vi "温湿度上位机.vi"() -> ()   [LabVIEW 2023]
uses:
  <vilib>/Instr/_visa.llb/VISA Configure Serial Port (Instr).vi
panel:
  out "传输次数":dbl
  out "湿度计":dbl(slide) scale=0.0..100.0
  out "温度计":dbl(slide) scale=0.0..100.0
  out "EE":string
  out "FF":string
  out "温度":dbl
  out "湿度":dbl
  out "读取字节数":u32
  out "VISA资源名称输出":refnum<visa-resource-name>
  out "read buffer":string
  out "send flag":bool
  in  "波特率":u64(ring) items=["9600"=9600, "115200"=115200]
  in  "停止":bool
  out "枚举":T1
  out "Serial state":bool
  in  "serial":refnum<visa-resource-name> caption="端口号"
  in  "打开串口":bool
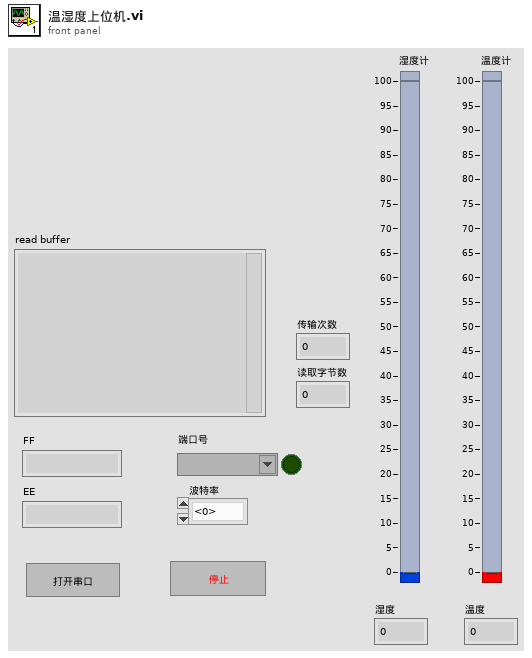
[diagram p1: front panel]
types:
  T1 = typedef "状态机.ctl" = enum16{"Init", "Wait", "GetData", "Send", "Deal", "Exit"}
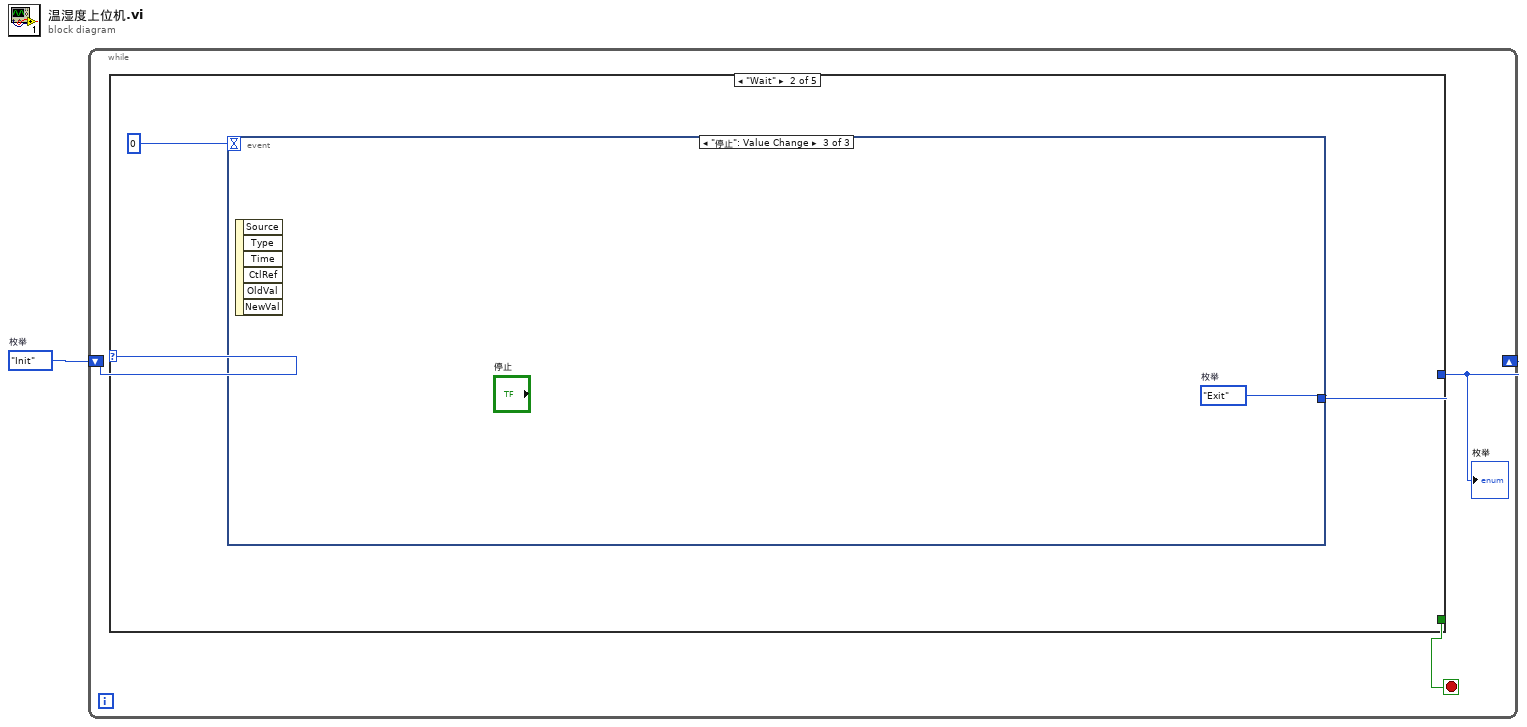
[diagram p0: block diagram]
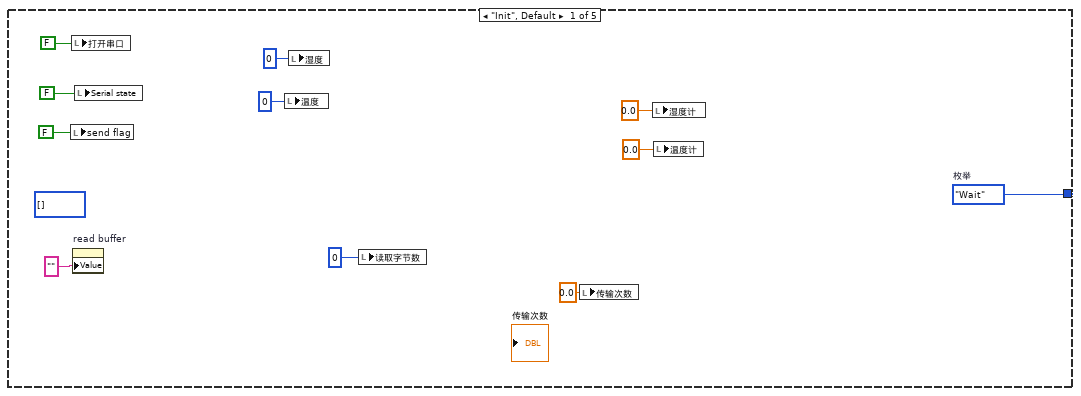
[diagram p2: hidden frame]
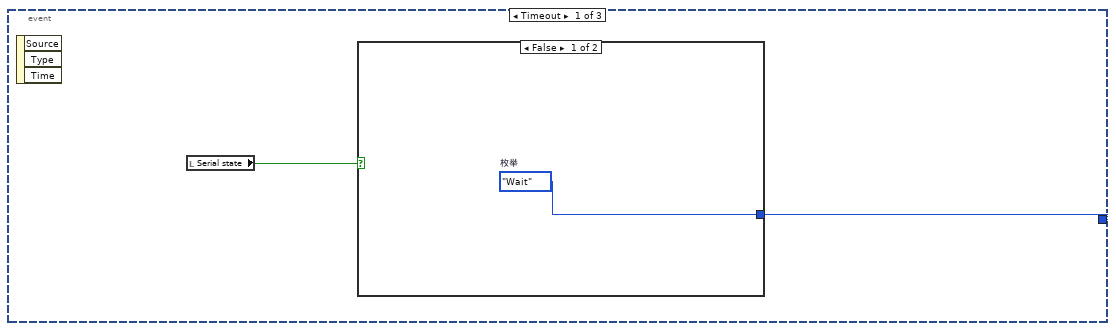
[diagram p3: hidden frame]
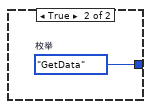
[diagram p4: hidden frame]
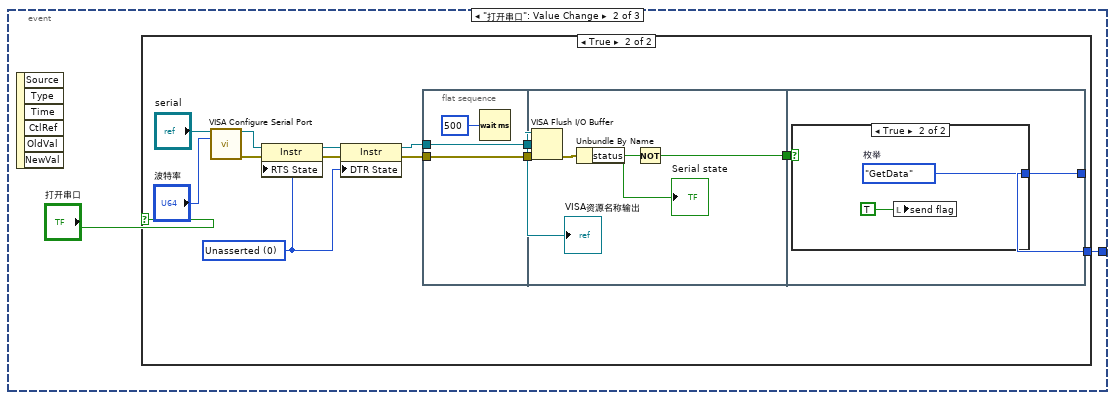
[diagram p5: hidden frame]
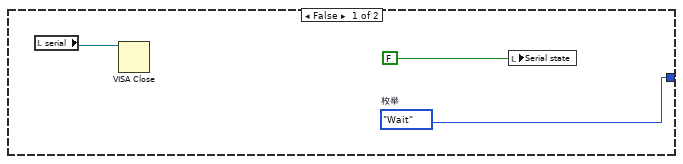
[diagram p6: hidden frame]
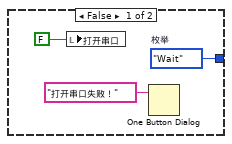
[diagram p7: hidden frame]
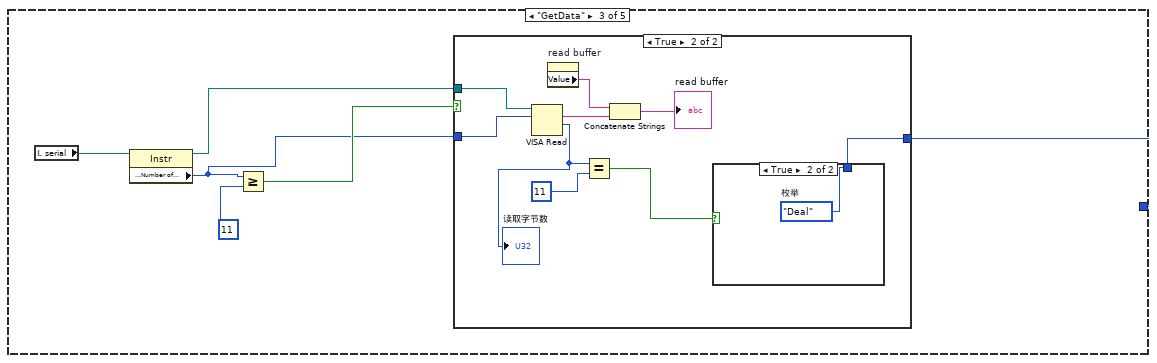
[diagram p8: hidden frame]
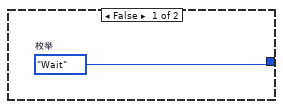
[diagram p9: hidden frame]
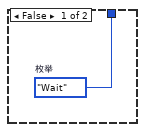
[diagram p10: hidden frame]
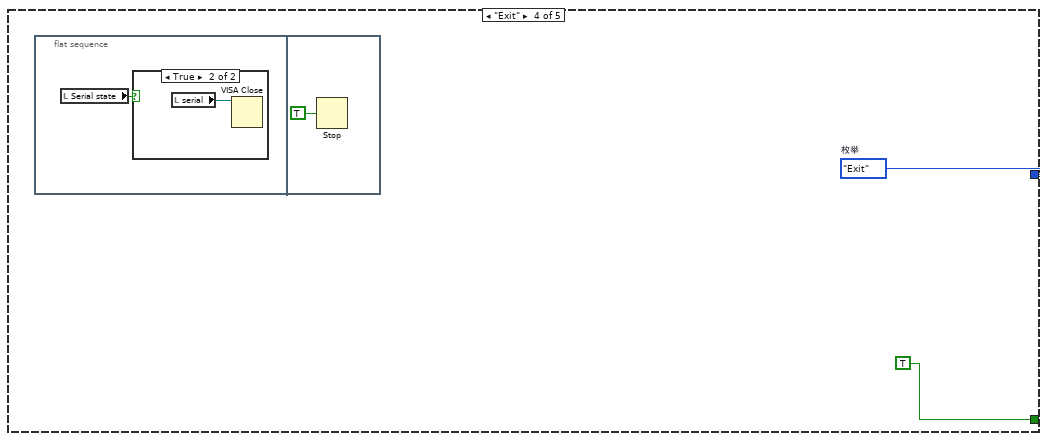
[diagram p11: hidden frame]
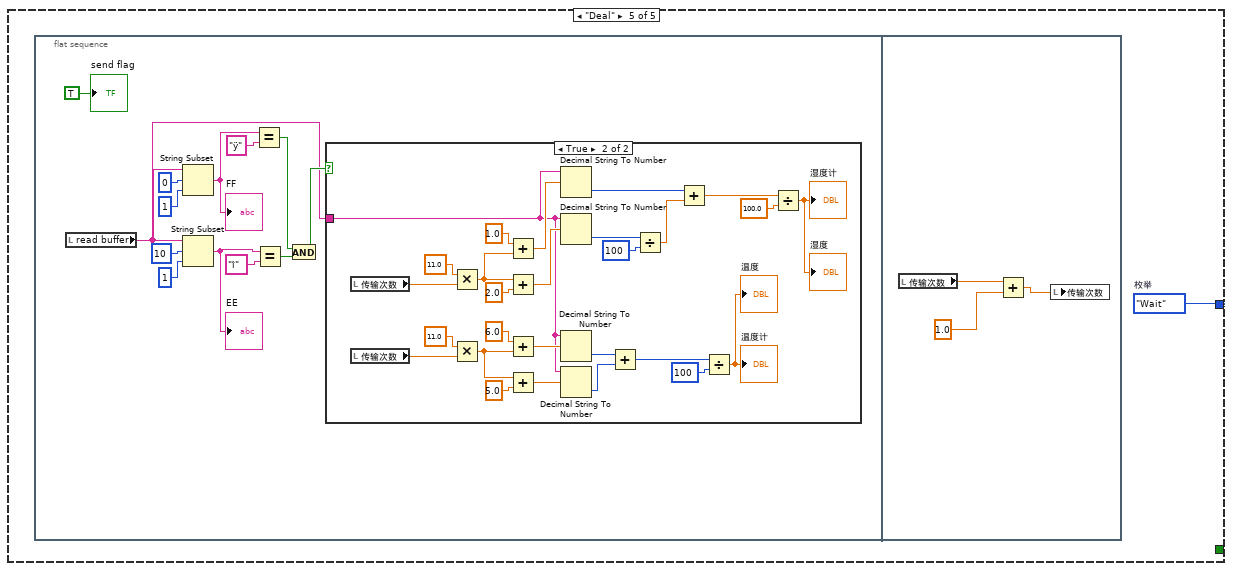
[diagram p13: hidden frame]
diagram:
  w1 = 状态机."Init"  # 枚举
  n1 = while {
    shift-right: [w3] -> _
    shift-left: w1 -> [w4]
    stop <- w2 stop-if-true
    n2 = case shown="\"Wait\"" w4 {
      tunnel: [w13 w16 w60 w76 w80] -> w3
      tunnel: [_ _ _ TRUE _] -> w2
      frame "Init", Default {
        (unwired) u32[] [] ("历史数据")
        w13 = 状态机."Wait"  # 枚举
        n3 = local write "send flag"(FALSE ("send flag")) -> ()
        n4 = local write "打开串口"(FALSE ("打开串口")) -> ()
        n5 = property on="read buffer" class="Str"("Value"="" ("read buffer")) -> ()  [unwired: 2 in, 2 out]
        n6 = local write "Serial state"(FALSE ("布尔")) -> ()
        n7 = local write "温度"(0 ("温度")) -> ()
        n8 = local write "湿度"(0 ("湿度")) -> ()
        n9 = local write "读取字节数"(u32 0 ("读取字节数")) -> ()
        n10 = local write "传输次数"(0.0 ("数值")) -> ()
        n11 = local write "湿度计"(0.0 ("湿度计")) -> ()
        n12 = local write "温度计"(0.0 ("温度计")) -> ()
      }
      frame "Wait" {
        n13 = event shown="[2] \"停止\": Value Change" {
          selector: _ -> [_ _ _]
          dyn-events: _ -> [_ _ _]
          timeout: 0 -> [_ _ _]
          tunnel: [w18 w22 w56] -> w16
          event Timeout {
            n14 = event-data() -> ()  [unwired: 1 in, 3 out]
            n15 = local read "Serial state"() -> (w19:bool)
            n16 = case shown="False" w19 {
              tunnel: [w20 w21] -> w18
              frame False {
                w20 = 状态机."Wait"  # 枚举
              }
              frame True {
                w21 = 状态机."GetData"  # 枚举
              }
            }
          }
          event "打开串口": Value Change {
            n17 = event-data() -> ()  [unwired: 1 in, 6 out]
            n18 = case shown="True" "打开串口" {
              tunnel: [w25 w27] -> w22
              frame False {
                w25 = 状态机."Wait"  # 枚举
                n19 = local read "serial"() -> (w24:refnum<visa-resource-name>)
                n20 = VISA Close(VISA resource name=w24) -> ()  [unwired: 1 in, 1 out]
                n21 = local write "Serial state"(FALSE ("布尔")) -> ()
              }
              frame True {
                w35 = i16 0 items=["Unknown"=-1, "Unasserted"=0, "Asserted"=1] ("Serial Settings:Modem Line Settings:Line DTR State")
                n22 = call-poly "VISA Configure Serial Port"("VISA resource name"="serial", "baud rate (9600)"="波特率") -> ("VISA resource name out"=w34:refnum<visa-resource-name>, "error out"=w33:errorcluster)  [unwired: 12 in]
                n23 = property class="Instr"(reference=w34, error in=w33, "RTS State"=w35) -> (reference out=w36:refnum<visa-resource-name>, error out=w37:errorcluster)
                n24 = property class="Instr"(reference=w36, error in=w37, "DTR State"=w35) -> (reference out=w32:refnum<visa-resource-name>, error out=w29:errorcluster)
                n25 = flat-sequence {
                  tunnel: w32 -> [w41]
                  tunnel: [w41] -> w31
                  tunnel: [w40] -> w30
                  tunnel: w29 -> [w40]
                  tunnel: w31 -> [w48]
                  tunnel: w30 -> [w44]
                  tunnel: [w45] -> w28
                  tunnel: w28 -> [w50]
                  tunnel: [w49] -> w27
                  frame #0 {
                    n26 = Wait (ms)(milliseconds to wait=u32 500 ("等待时间（毫秒）")) -> ()  [unwired: 1 out]
                  }
                  frame #1 {
                    n27 = VISA Flush I/O Buffer(VISA resource name=w48, error in (no error)=w44) -> (VISA resource name out=→"VISA资源名称输出":refnum<visa-resource-name>, error out=w46:errorcluster)  [unwired: 1 in]
                    n28 = Unbundle By Name(w46) -> ("status"=w47:bool)
                    n29 = Not(x=w47) -> (.not. x?=w45:bool)
                    "Serial state" <- w45
                  }
                  frame #2 {
                    n30 = case shown="True" w50 {
                      tunnel: [w51 w55] -> w49
                      frame False {
                        w51 = 状态机."Wait"  # 枚举
                        n31 = local write "打开串口"(FALSE ("打开串口")) -> ()
                        n32 = One Button Dialog(message="打开串口失败！" ("消息")) -> ()  [unwired: 1 in, 1 out]
                      }
                      frame True {
                        w55 = 状态机."GetData"  # 枚举
                        n33 = local write "send flag"(TRUE ("send flag")) -> ()
                      }
                    }
                  }
                }
              }
            }
          }
          event "停止": Value Change {
            w56 = 状态机."Exit"  # 枚举
            n34 = event-data() -> ()  [unwired: 1 in, 6 out]
          }
        }
      }
      frame "GetData" {
        n35 = local read "serial"() -> (w62:refnum<visa-resource-name>)
        n36 = property class="Instr"(reference=w62) -> (reference out=w61:refnum<visa-resource-name>, "Serial Settings:Number of Bytes at Serial Port"=w58:u32)  [unwired: 1 in, 1 out]
        n37 = Greater Or Equal?(x=w58, y=u32 11) -> (x >= y?=w59:bool)
        n38 = case shown="True" w59 {
          tunnel: w61 -> [_ w72]
          tunnel: w58 -> [_ w71]
          tunnel: [w63 w67] -> w60
          frame False {
            w63 = 状态机."Wait"  # 枚举
          }
          frame True {
            n39 = VISA Read(VISA resource name=w72, byte count=w71) -> (read buffer=w66:string, return count=w70:u32)  [unwired: 1 in, 2 out]
            "读取字节数" <- w70
            n40 = property on="read buffer" class="Str"() -> ("Value"=w64:string)  [unwired: 2 in, 2 out]
            n41 = Equal?(x=w70, y=u32 11) -> (x = y?=w68:bool)
            n42 = Concatenate Strings(w64, w66) -> (→"read buffer":string)
            n43 = case shown="True" w68 {
              tunnel: [w73 w74] -> w67
              frame False {
                w73 = 状态机."Wait"  # 枚举
              }
              frame True {
                w74 = 状态机."Deal"  # 枚举
              }
            }
          }
        }
      }
      frame "Exit" {
        w76 = 状态机."Exit"  # 枚举
        n44 = flat-sequence {
          frame #0 {
            n45 = local read "Serial state"() -> (w77:bool)
            n46 = case shown="True" w77 {
              frame False {
              }
              frame True {
                n47 = local read "serial"() -> (w78:refnum<visa-resource-name>)
                n48 = VISA Close(VISA resource name=w78) -> ()  [unwired: 1 in, 1 out]
              }
            }
          }
          frame #1 {
            n49 = Stop(stop? (T)=TRUE ("停止？(T)")) -> ()
          }
        }
      }
      frame "Deal" {
        w80 = 状态机."Wait"  # 枚举
        n50 = flat-sequence {
          frame #0 {
            n51 = local read "read buffer"() -> (w81:string)
            n52 = String Subset(string=w81, offset (0)=0 ("偏移量(0)"), length (rest)=1 ("长度（剩余）")) -> (substring=w89:string)
            "FF" <- w89
            n53 = String Subset(string=w81, offset (0)=10 ("偏移量(0)"), length (rest)=1 ("长度（剩余）")) -> (substring=w88:string)
            "EE" <- w88
            n54 = Equal?(x=w89, y="ÿ") -> (x = y?=w82:bool)
            n55 = Equal?(x=w88, y="î") -> (x = y?=w84:bool)
            n56 = And(x=w82, y=w84) -> (x .and. y?=w83:bool)
            n57 = case shown="True" w83 {
              tunnel: w81 -> [_ w95]
              frame False {
              }
              frame True {
                n58 = local read "传输次数"() -> (w117:dbl)
                n59 = local read "传输次数"() -> (w113:dbl)
                n60 = Multiply(x=11.0, y=w117) -> (x*y=w111:dbl)
                n61 = Multiply(x=11.0, y=w113) -> (x*y=w100:dbl)
                n62 = Add(x=1.0, y=w111) -> (x+y=w120:dbl)
                n63 = Add(x=w111, y=2.0) -> (x+y=w112:dbl)
                n64 = Add(x=6.0, y=w100) -> (x+y=w116:dbl)
                n65 = Add(x=w100, y=5.0) -> (x+y=w102:dbl)
                n66 = Decimal String To Number(string=w95, offset=w120) -> (number=w106:i32)  [unwired: 1 in, 1 out]
                n67 = Decimal String To Number(string=w95, offset=w112) -> (number=w109:i32)  [unwired: 1 in, 1 out]
                n68 = Decimal String To Number(string=w95, offset=w116) -> (number=w94:i32)  [unwired: 1 in, 1 out]
                n69 = Decimal String To Number(string=w95, offset=w102) -> (number=w96:i32)  [unwired: 1 in, 1 out]
                n70 = Add(x=w94, y=w96) -> (x+y=w99:i32)
                n71 = Divide(x=w109, y=100) -> (x/y=w107:dbl)
                n72 = Add(x=w106, y=w107) -> (x+y=w105:dbl)
                n73 = Divide(x=w99, y=100) -> (x/y=→"温度" →"温度计":dbl)
                n74 = Divide(x=w105, y=100.0) -> (x/y=→"湿度" →"湿度计":dbl)
              }
            }
            "send flag" <- TRUE ("send flag")
          }
          frame #1 {
            n75 = local read "传输次数"() -> (w123:dbl)
            n76 = Add(x=w123, y=1.0) -> (x+y=w121:dbl)
            n77 = local write "传输次数"(w121) -> ()
          }
        }
      }
    }
    "枚举" <- w3
  }
